vi "Test Write and Read Data.vi"() -> ()   [LabVIEW 2019]
uses:
  <vilib>/Analysis/1siggen.llb/Ramp Pattern by Samples.vi
  src/LV-Data.PG/API/Write Variable (one-row).vi
  src/LV-Data.PG/API/Read Variable (double).vi
  src/LV-Data.PG/LV-Data.PGSQL.lvclass
  <vilib>/Analysis/NI_AALBase.lvlib
panel:
  out "Wrote to DB?":bool
  out "XY Graph 2":cluster{timestamp[], dbl[]}(graph)
  out "XY Graph":cluster{timestamp[], dbl[]}(graph)
  in  "stop":bool
  in  "single (F = multirows)":bool
  out "Read Cluster":T1
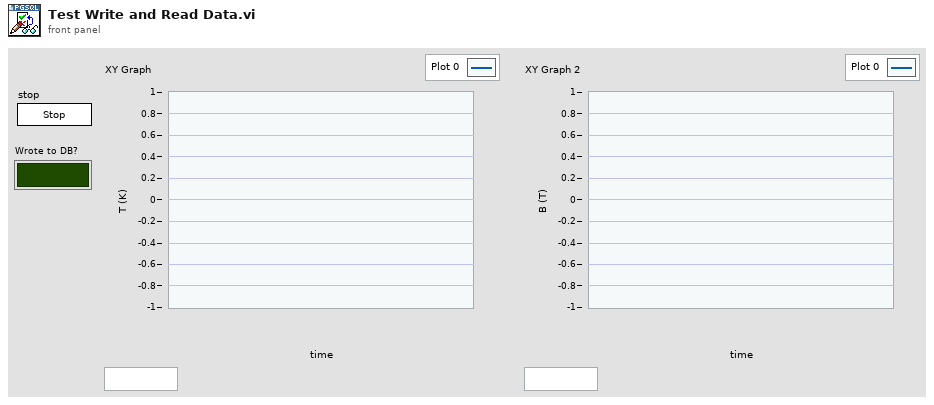
[diagram p1: front panel]
types:
  T1 = cluster{"Value":dbl, "Value":dbl, "Value":string, "Value":bool}
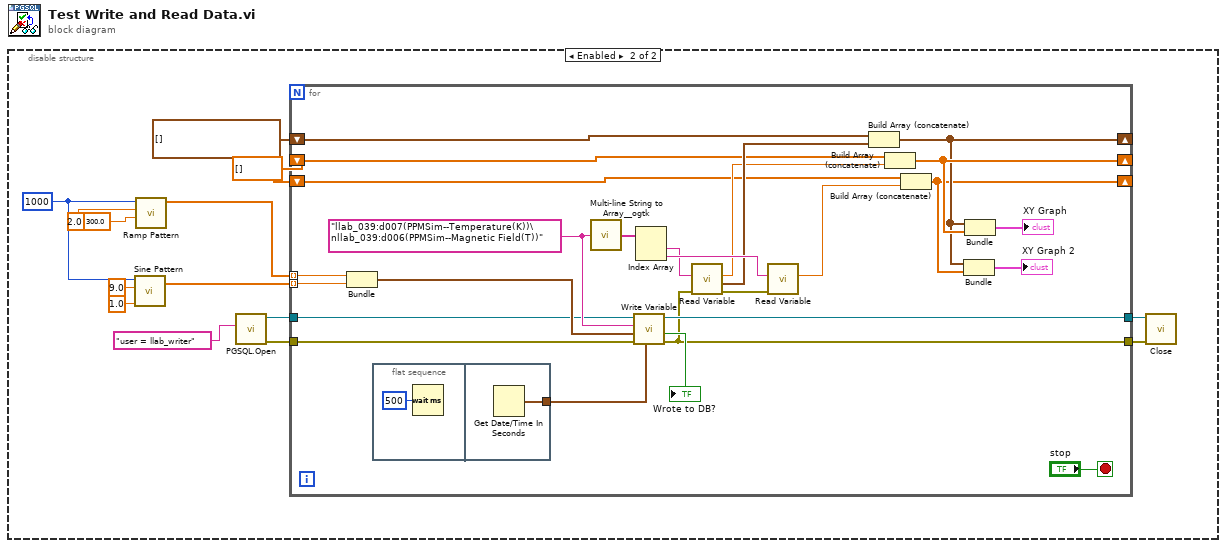
[diagram p0: block diagram]
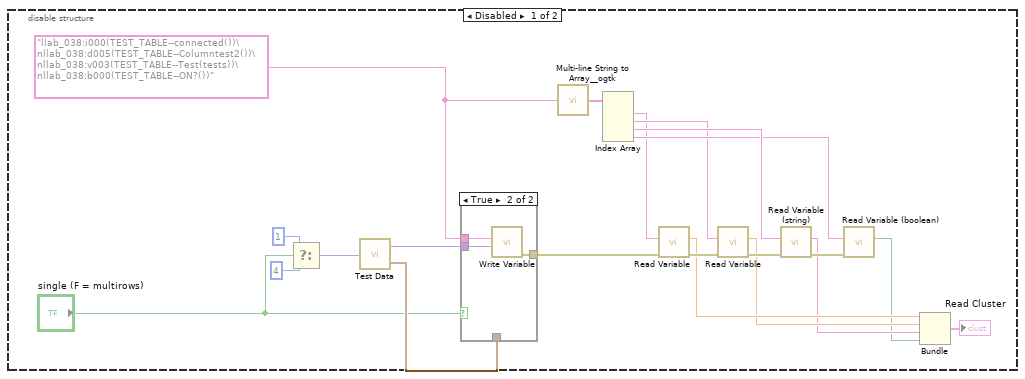
[diagram p2: hidden frame]
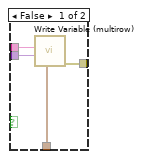
[diagram p3: hidden frame]
diagram:
  n1 = disable-structure shown="Enabled" {
    frame Disabled {
      w21 = "llab_038:i000(TEST_TABLE--connected())\nllab_038:d005(TEST_TABLE--Columntest2())\nllab_038:v003(TEST_TABLE--Test(tests))\nllab_038:b000(TEST_TABLE--ON?())" ("variable")
      n2 = Select(t=1, s="single (F = multirows)", f=4 ("Size")) -> (s? t:f=w20:i32)
      n3 = call "Test Data.vi"("Size"=w20) -> ("Data"=w4:variant, "Timestamps"=w5:timestamp[])
      n4 = case shown="True" "single (F = multirows)" {
        tunnel: w21 -> [w22 w28]
        tunnel: [w25 w27] -> w19
        tunnel: w5 -> [w24 _]
        tunnel: w4 -> [w23 w26]
        frame False {
          n5 = call "Write Variable (multirow).vi"("Time Stamps"=w24, "Data"=w23, "Path(s)"=w22) -> ("error out"=w25:errorcluster)  [unwired: 5 in, 3 out]
        }
        frame True {
          n6 = call-poly "Write Variable.vi"("Data"=w26, "variable"=w28) -> ("error out"=w27:errorcluster)  [unwired: 6 in, 3 out]
        }
      }
      n7 = call <userlib>:"Multi-line String to Array__ogtk.vi"("string"=w21) -> ("lines"=w15:string[])
      n8 = Index Array(array=w15) -> (element #1=w11:string, element #2=w12:string, element #3=w14:string, element #4=w13:string)  [unwired: 4 in]
      n9 = call-poly "Read Variable.vi"("error in (no error)"=w19, "PG path"=w11) -> ("error out"=w18:errorcluster, "Value"=w10:dbl)  [unwired: 6 in, 2 out]
      n10 = call-poly "Read Variable.vi"("error in (no error)"=w18, "PG path"=w12) -> ("error out"=w17:errorcluster, "Value"=w9:dbl)  [unwired: 6 in, 2 out]
      n11 = call "Read Variable (string).vi"("error in (no error)"=w17, "PG path"=w14) -> ("error out"=w16:errorcluster, "Value"=w8:string)  [unwired: 4 in, 4 out]
      n12 = call "Read Variable (boolean).vi"("error in (no error)"=w16, "PG path"=w13) -> ("Value"=w7:bool)  [unwired: 4 in, 5 out]
      n13 = Bundle("Value"=w10, "Value"=w9, "Value"=w8, "Value"=w7) -> (→"Read Cluster":T1)  [unwired: 1 in]
    }
    frame Enabled {
      w34 = dbl[] []
      w42 = 1000 ("samples")
      n14 = call <vilib>:"Sine Pattern.vi"("cycles"=1.0, "amplitude"=9.0, "samples"=w42) -> ("Sinusoidal Pattern"=w36:dbl[])  [unwired: 1 in, 1 out]
      n15 = call-poly <vilib>:"Ramp Pattern.vi"("start"=300.0, "end"=2.0, "samples"=w42) -> ("Ramp Pattern"=w37:dbl[])  [unwired: 7 in, 1 out]
      n16 = call "PGSQL.Open.vi"("Connection String"="user = llab_writer") -> ("error out"=w30:errorcluster, "Data.PG out"=w33:refnum<class "LV-Data.PGSQL.lvclass">)  [unwired: 9 in]
      n17 = for {
        tunnel: w37 -> [w63] mode=indexing
        tunnel: w36 -> [w62] mode=indexing
        shift-right: [w51] -> _
        shift-left: timestamp[] [] -> [w54]
        shift-right: [w52] -> _
        shift-left: w34 -> [w53]
        shift-right: [w50] -> _
        shift-left: w34 -> [w55]
        tunnel: w33 -> [w46]
        tunnel: [w45] -> w32
        tunnel: [w44] -> w31
        tunnel: w30 -> [w43]
        stop <- "stop" stop-if-true
        w68 = "llab_039:d007(PPMSim--Temperature(K))\nllab_039:d006(PPMSim--Magnetic Field(T))" ("variable")
        n18 = Bundle(w63, w62) -> (w60:cluster{dbl, dbl})  [unwired: 1 in]
        n19 = flat-sequence {
          tunnel: [w70] -> w61
          frame #0 {
            n20 = Wait (ms)(milliseconds to wait=u32 500) -> ()  [unwired: 1 out]
          }
          frame #1 {
            n21 = Get Date/Time In Seconds() -> (seconds since 1Jan1904=w70:timestamp)
          }
        }
        n22 = call <userlib>:"Multi-line String to Array__ogtk.vi"("string"=w68) -> ("lines"=w66:string[])
        n23 = call-poly "Write Variable.vi"("Time Stamp"=w61, "error in (no error)"=w43, "Data"=w60, "variable"=w68, "Data.PG in"=w46) -> ("error out"=w44:errorcluster, "Wrote to DB?"=→"Wrote to DB?":bool, "Data.PG out"=w45:refnum<class "LV-Data.PGSQL.lvclass">)  [unwired: 3 in, 1 out]
        n24 = Index Array(array=w66) -> (element #1=w64:string, element #2=w65:string)  [unwired: 2 in]
        n25 = call-poly "Read Variable.vi"("error in (no error)"=w44, "PG path"=w64) -> ("error out"=w67:errorcluster, "Time Stamp"=w58:timestamp, "Value"=w57:dbl)  [unwired: 6 in, 1 out]
        n26 = call-poly "Read Variable.vi"("error in (no error)"=w67, "PG path"=w65) -> ("Value"=w56:dbl)  [unwired: 6 in, 3 out]
        n27 = Build Array (concatenate)(w54, w58) -> (w51:timestamp[])
        n28 = Build Array (concatenate)(w53, w57) -> (w52:dbl[])
        n29 = Build Array (concatenate)(w55, w56) -> (w50:dbl[])
        n30 = Bundle(w51, w50) -> (→"XY Graph 2":cluster{timestamp[], dbl[]})  [unwired: 1 in]
        n31 = Bundle(w51, w52) -> (→"XY Graph":cluster{timestamp[], dbl[]})  [unwired: 1 in]
      }
      n32 = call-dynamic "Close.vi"("error in (no error)"=w31, "Data.PG in"=w32) -> ()  [unwired: 8 in, 2 out]
    }
  }
